vi "Write Log command_.vi"(10 "Log command?":bool=TRUE, 11 "Generic UI Process Command in":refnum<class "Generic UI Process Command.lvclass">) -> (3 "Generic UI Process Command out":refnum<class "Generic UI Process Command.lvclass">)   [LabVIEW 2019, in "User Interface Process.lvlib" / "Generic UI Process Command.lvclass"]
uses:
  Generic UI Process Command.lvclass
  Generic UI Process Command.lvclass/Generic UI Process Command.ctl
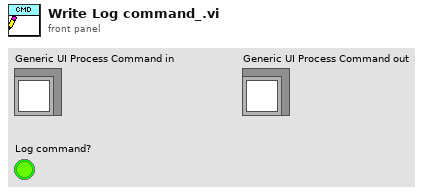
[diagram p1: front panel]
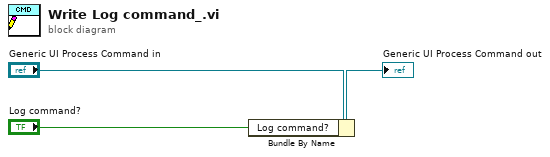
[diagram p0: block diagram]
diagram:
  n1 = Bundle By Name(cluster="Generic UI Process Command in", "Log command?"="Log command?") -> (→"Generic UI Process Command out":refnum<class "Generic UI Process Command.lvclass">)
